vi "AlliGator Convert Decay Fit Options v3 to v4.vi"(1 "Decay Fit Options (v3)":T1 {"Confidence Level" min=0.0 max=100.0; "Offset Resolution" min=0.0; "Period" min=0.0; "Min Decay Percentile" min=0.0 max=1.0; "Max Decay Percentile" min=0.0 max=100.0}) -> (0 "Decay Fit Options (v4)":T8 {"Confidence Level" min=0.0 max=100.0; "Offset Resolution" min=0.0; "Period" min=0.0; "Min Decay Percentile" min=0.0 max=1.0; "Max Decay Percentile" min=0.0 max=100.0})   [LabVIEW 2021, in "AlliGator Decay Fit Parameter Map.lvlib"]
uses:
  AlliGator Decay Fit Parameter Map.lvlib
  Fits/Decay Convolution/Decay Model.ctl
  Fits/Fits.lvlib
  Fits/Residual Type.ctl
  Fits/IRF(X)PSED/Fit Weights Type v2.ctl
  Fits/Non-linear Fitting Method v2.ctl
  Fits/Fit Calculation Method.ctl
  Fits/Non-linear Fitting Algorithm.ctl
  Fits/IRF(X)PSED/Decay Fit Options v4.ctl
  Fits/IRF(X)PSED/Fit Weights Type.ctl
  Fits/IRF(X)PSED/Decay Fit Options v3.ctl
panel:
  # "see the License on the block diagram (Ctrl+E or Window:Show Block Diagram)"
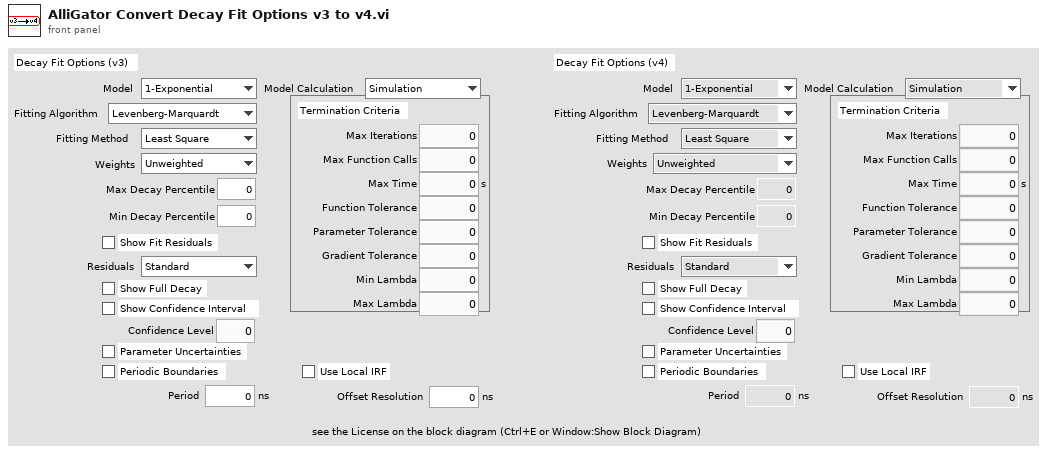
[diagram p1: front panel]
types:
  T1 = typedef "Fits.lvlib/Decay Fit Options v3.ctl" = cluster{"Show Fit Residuals":bool, "Fit Model":T2, "Residual Type":T3, "Max Decay Percentile":dbl, "Min Decay Percentile":dbl, "Show Full Decay":bool, "Weights":T4, "Fitting Method":T5, "Compute Parameter Uncertainties":bool, "Periodic Boundaries":bool, "Model Calculation":T6, "Period":dbl[unit], "Termination Criteria":cluster{"Max Iterations":i32, "Max Function Calls":i32, "Max Time":dbl[unit], "Function Tolerance":dbl, "Parameter Tolerance":dbl, "Gradient Tolerance":dbl, "Min Lambda":dbl, "Max Lambda":dbl, "Initial Tick Count":u32}, "Offset Resolution":dbl[unit], "Use Local IRF":bool, "Fitting Algorithm":T7, "Show Confidence Interval ":bool, "Confidence Level":dbl}
  T2 = typedef "Fits.lvlib/Decay Model.ctl" = enum16{"1-Exponential", "2-Exponentials"}
  T3 = typedef "Fits.lvlib/Residual Type.ctl" = enum16{"Standard", "Normalized", "Reduced"}
  T4 = typedef "Fits.lvlib/Fit Weights Type.ctl" = enum16{"Unweighted", "1/Variance", "Best of All"}
  T5 = typedef "Fits.lvlib/Non-linear Fitting Method v2.ctl" = enum16{"Least Square", "Least Absolute Residual", "Bisquare", "MLE", "-", "Best of All"}
  T6 = typedef "Fits.lvlib/Fit Calculation Method.ctl" = enum16{"Simulation", "Convolution", "Integration"}
  T7 = typedef "Fits.lvlib/Non-linear Fitting Algorithm.ctl" = enum16{"Levenberg-Marquardt", "Trust-Region Dogleg"}
  T8 = typedef "Fits.lvlib/Decay Fit Options v4.ctl" = cluster{"Show Fit Residuals":bool, "Fit Model":T2, "Residual Type":T3, "Max Decay Percentile":dbl, "Min Decay Percentile":dbl, "Show Full Decay":bool, "Weights":T9, "Fitting Method":T5, "Compute Parameter Uncertainties":bool, "Periodic Boundaries":bool, "Model Calculation":T6, "Period":dbl[unit], "Termination Criteria":cluster{"Max Iterations":i32, "Max Function Calls":i32, "Max Time":dbl[unit], "Function Tolerance":dbl, "Parameter Tolerance":dbl, "Gradient Tolerance":dbl, "Min Lambda":dbl, "Max Lambda":dbl, "Initial Tick Count":u32}, "Offset Resolution":dbl[unit], "Use Local IRF":bool, "Fitting Algorithm":T7, "Show Confidence Interval ":bool, "Confidence Level":dbl}
  T9 = typedef "Fits.lvlib/Fit Weights Type v2.ctl" = enum16{"Unweighted", "1/Variance (Neyman)", "1/Variance (Pearson)", "Best of All"}
  T10 = cluster{"Max Iterations":i32, "Max Function Calls":i32, "Max Time":dbl[unit], "Function Tolerance":dbl, "Parameter Tolerance":dbl, "Gradient Tolerance":dbl, "Min Lambda":dbl, "Max Lambda":dbl, "Initial Tick Count":u32}
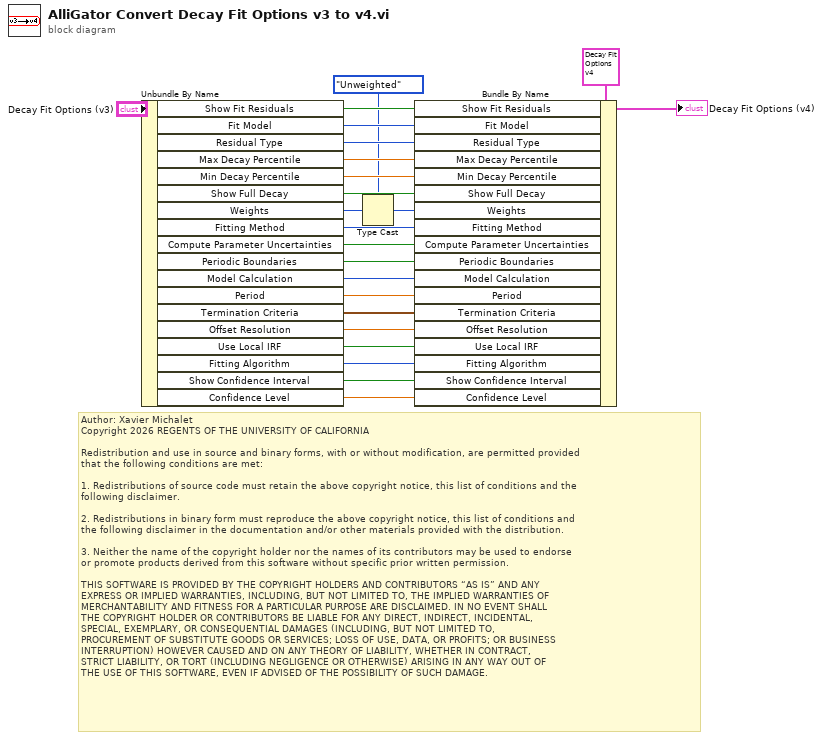
[diagram p0: block diagram]
diagram:
  # "Author: Xavier Michalet\nCopyright 2026 REGENTS OF THE UNIVERSITY OF CALIFORNIA\n\nRedistribution and use in source and binary forms, with or without modification, are permitted provided\nthat the following conditions are met:\n\n1. Redistributions of source code must retain the above copyright notice, this list of conditions and the\nfollowing disclaimer.\n\n2. Redistributions in binary form must reproduce the above copyright notice, this list of conditions and\nthe following disclaimer in the documentation and/or other materials provided with the distribution.\n\n3. Neither the name of the copyright holder nor the names of its contributors may be used to endorse \nor promote products derived from this software without specific prior written permission.\n\nTHIS SOFTWARE IS PROVIDED BY THE COPYRIGHT HOLDERS AND CONTRIBUTORS “AS IS” AND ANY \nEXPRESS OR IMPLIED WARRANTIES, INCLUDING, BUT NOT LIMITED TO, THE IMPLIED WARRANTIES OF\nMERCHANTABILITY AND FITNESS FOR A PARTICULAR PURPOSE ARE DISCLAIMED. IN NO EVENT SHALL\nTHE COPYRIGHT HOLDER OR CONTRIBUTORS BE LIABLE FOR ANY DIRECT, INDIRECT, INCIDENTAL, \nSPECIAL, EXEMPLARY, OR CONSEQUENTIAL DAMAGES (INCLUDING, BUT NOT LIMITED TO, \nPROCUREMENT OF SUBSTITUTE GOODS OR SERVICES; LOSS OF USE, DATA, OR PROFITS; OR BUSINESS\nINTERRUPTION) HOWEVER CAUSED AND ON ANY THEORY OF LIABILITY, WHETHER IN CONTRACT, \nSTRICT LIABILITY, OR TORT (INCLUDING NEGLIGENCE OR OTHERWISE) ARISING IN ANY WAY OUT OF\nTHE USE OF THIS SOFTWARE, EVEN IF ADVISED OF THE POSSIBILITY OF SUCH DAMAGE."
  n1 = Unbundle By Name("Decay Fit Options (v3)") -> ("Show Fit Residuals"=w19:bool, "Fit Model"=w18:T2, "Residual Type"=w17:T3, "Min Decay Percentile"=w16:dbl, "Show Full Decay"=w15:bool, "Weights"=w14:T4, "Fitting Method"=w11:T5, "Compute Parameter Uncertainties"=w10:bool, "Periodic Boundaries"=w9:bool, "Model Calculation"=w8:T6, "Period"=w7:dbl[unit], "Termination Criteria"=w6:T10, "Offset Resolution"=w5:dbl[unit], "Use Local IRF"=w4:bool, "Fitting Algorithm"=w3:T7, "Show Confidence Interval"=w2:bool, "Confidence Level"=w1:dbl)  [unwired: 1 out]
  n2 = Type Cast(type=Fit_Weights_Type_v2."Unweighted" ("Weights"), x=w14) -> (*(type *) &x=w13:T9)
  n3 = Bundle By Name(cluster=T8 {"Show Fit Residuals"=FALSE, "Fit Model"=enum."1-Exponential", "Residual Type"=enum."Standard", "Max Decay Percentile"=0.0, "Min Decay Percentile"=0.0, "Show Full Decay"=FALSE, "Weights"=enum."Unweighted", "Fitting Method"=enum."Least Square", "Compute Parameter Uncertainties"=FALSE, "Periodic Boundaries"=FALSE, "Model Calculation"=enum."Simulation", "Period"=0.0, "Termination Criteria"={"Max Iterations"=0, "Max Function Calls"=0, "Max Time"=0.0, "Function Tolerance"=0.0, "Parameter Tolerance"=0.0, "Gradient Tolerance"=0.0, "Min Lambda"=0.0, "Max Lambda"=0.0, "Initial Tick Count"=0}, "Offset Resolution"=0.0, "Use Local IRF"=FALSE, "Fitting Algorithm"=enum."Levenberg-Marquardt", "Show Confidence Interval "=FALSE, "Confidence Level"=0.0} ("Decay Fit Options (v4)"), "Show Fit Residuals"=w19, "Fit Model"=w18, "Residual Type"=w17, "Max Decay Percentile"=w16, "Min Decay Percentile"=w16, "Show Full Decay"=w15, "Weights"=w13, "Fitting Method"=w11, "Compute Parameter Uncertainties"=w10, "Periodic Boundaries"=w9, "Model Calculation"=w8, "Period"=w7, "Termination Criteria"=w6, "Offset Resolution"=w5, "Use Local IRF"=w4, "Fitting Algorithm"=w3, "Show Confidence Interval"=w2, "Confidence Level"=w1) -> (→"Decay Fit Options (v4)":T8)
